vi "Load_Cache.vi"(8 "error in (no error)":errorcluster, 11 "AB_Build in":refnum<class "AB_Build.lvclass">) -> (0 "error out":errorcluster, 2 "valid format?":bool, 3 "AB_Build out":refnum<class "AB_Build.lvclass">)   [LabVIEW 2020, in "AB_Build.lvclass"]
uses:
  <vilib>/AppBuilder/AB_Classes/Build/AB_Build.lvclass
  <vilib>/AppBuilder/AB_Classes/Build/AB_Build.lvclass/AB_Build.ctl
  <vilib>/AppBuilder/RW_Project/AB_RW_Project_PropBag_Action.ctl
  <vilib>/AppBuilder/AB_Classes/PreviewCache/PreviewCache.lvclass
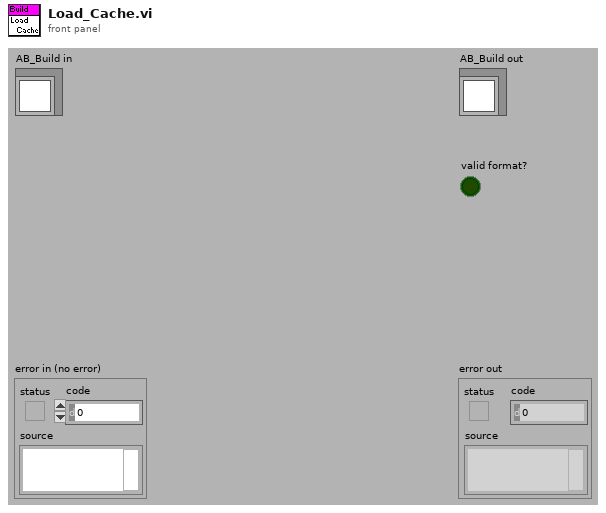
[diagram p1: front panel]
types:
  T1 = typedef "AB_RW_Project_PropBag_Action.ctl" = enum16{"read", "write", "clear", "readPrevious", "writePrevious", "clearPrevious"}
  T2 = typedef "ItemRef.ctl" = u64
  T3 = typedef "AB_RW_Project_Cache_Data.ctl" = cluster{"build preview data":T4, "project symbol checksum":string, "target symbol checksum":string, "My Computer checksum":string}
  T4 = typedef "build preview data.ctl" = cluster{"generated files":path[], "output directory":path, "buildVersion":cluster{"major":u16, "minor":u16, "patch":u16, "build":u16}}
  T5 = typedef "PreviewCache.ctl" = cluster{"build preview data":T4, "project symbol checksum":string, "target symbol checksum":string, "My Computer checksum":string}
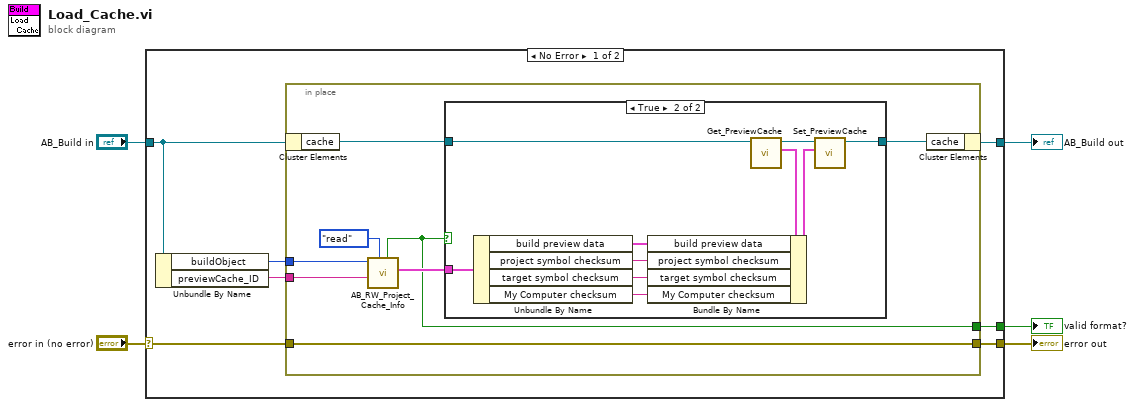
[diagram p0: block diagram]
diagram:
  n1 = case shown="No Error" "error in (no error)" {
    selector: "error in (no error)" -> [w9 w33]
    tunnel: [w8 w33] -> w4
    tunnel: [w12 w32] -> w2
    tunnel: "AB_Build in" -> [w11 w32]
    tunnel: [w6 _] -> w1
    frame No Error {
      n2 = Unbundle By Name(w11) -> ("buildObject"=w10:T2, "previewCache_ID"=w7:string)
      n3 = in-place {
        in-place-border: w10 -> [w16]
        in-place-border: w9 -> [w15]
        in-place-border: [w15] -> w8
        in-place-border: w7 -> [w14]
        in-place-border: [w13] -> w6
        n4 = in-place-cluster #1(w11) -> ("cache"=w17:refnum<class "PreviewCache.lvclass">)
        n5 = call <vilib>:"AB_RW_Project_Cache_Info.vi"("action"=AB_RW_Project_PropBag_Action."read", "cache_ID"=w14, "Object In"=w16) -> ("info out"=w19:T3, "valid format?"=w13:bool)  [unwired: 4 in, 3 out]
        n6 = case shown="True" w13 {
          tunnel: w19 -> [_ w30]
          tunnel: [w21 w24] -> w18
          tunnel: w17 -> [w21 w23]
          frame False {
          }
          frame True {
            n7 = Unbundle By Name(w30) -> ("build preview data"=w28:T4, "project symbol checksum"=w25:string, "target symbol checksum"=w27:string, "My Computer checksum"=w26:string)
            n8 = call <vilib>:"Get_PreviewCache.vi"("PreviewCache in"=w23) -> ("data"=w22:T5, "PreviewCache out"=w31:refnum<class "PreviewCache.lvclass">)  [unwired: 8 in, 1 out]
            n9 = Bundle By Name(cluster=w22, "build preview data"=w28, "project symbol checksum"=w25, "target symbol checksum"=w27, "My Computer checksum"=w26) -> (w29:T5)
            n10 = call <vilib>:"Set_PreviewCache.vi"("data"=w29, "PreviewCache in"=w31) -> ("PreviewCache out"=w24:refnum<class "PreviewCache.lvclass">)  [unwired: 8 in, 1 out]
          }
        }
        n11 = in-place-cluster #1("cache"=w18) -> (w12:refnum<class "AB_Build.lvclass">)
      }
    }
    frame Error {
    }
  }
  "error out" <- w4
  "AB_Build out" <- w2
  "valid format?" <- w1
